vi "JSONconfig.vi"(2 "error in (no error)":errorcluster, 3 "file path (use dialog)":path, 4 "config file inputs":T5 {"Oscilloscope Configuration Input Array"."vertical coupling" items=["AC", "DC", "Ground"]}) -> (0 "error out":errorcluster, 1 "Instrument Configuration Clusters":T4 {"Oscilloscope Configuration Input Array"."vertical coupling" items=["AC", "DC", "Ground"]})   [LabVIEW 2019]
uses:
  Controls/VISA_power_Control.ctl
  Controls/RFBlockControl.ctl
  <instrlib>/niScope/Controls/niScope vertical coupling.ctl
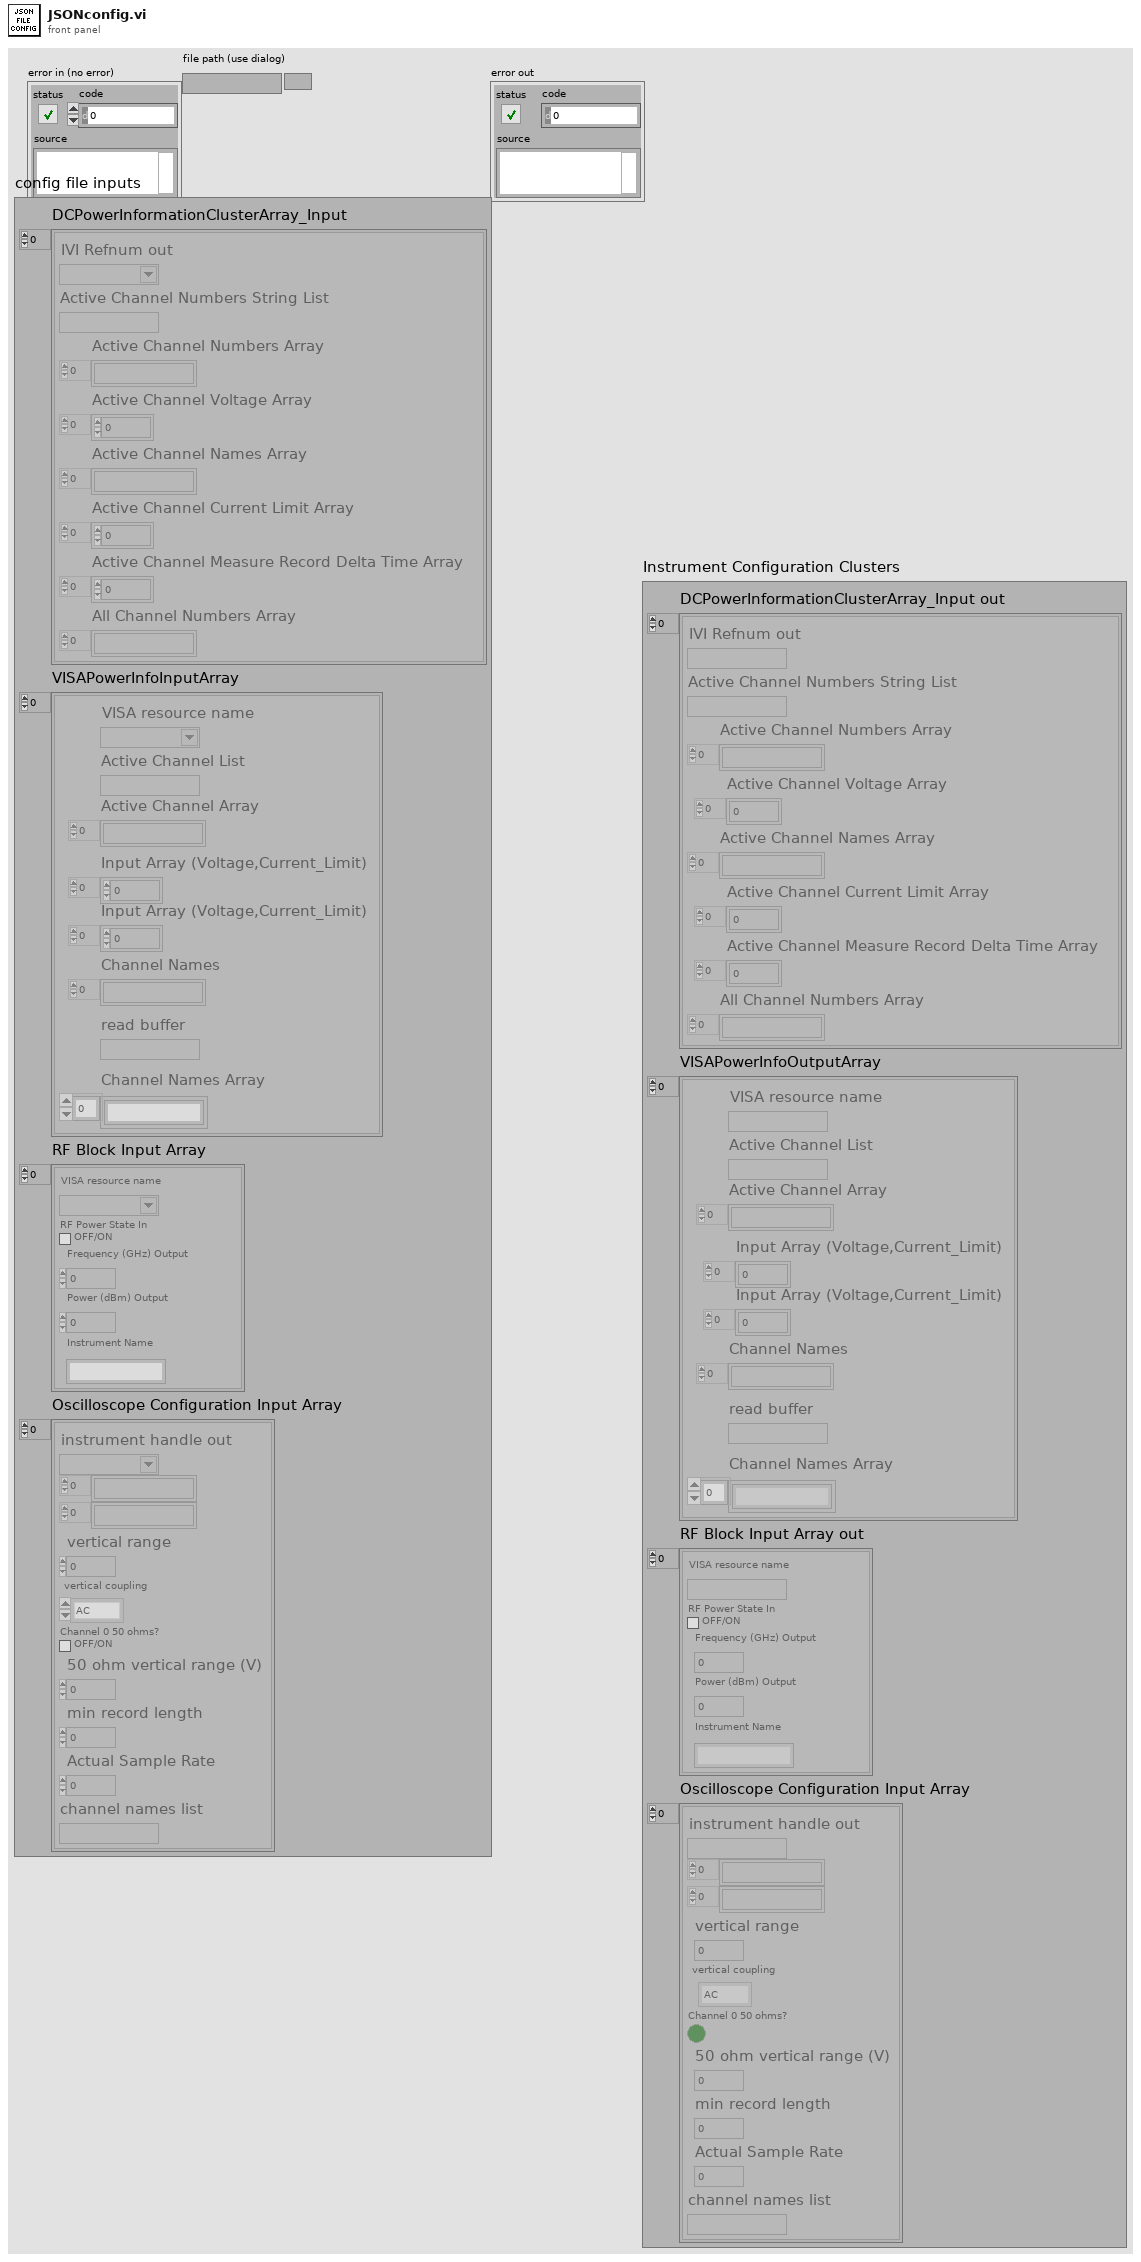
[diagram p1: front panel]
types:
  T1 = typedef "VISA_power_Control.ctl" = cluster{"VISA resource name":refnum<visa-resource-name>, "Active Channel List":string, "Active Channel Array":string[], "Input Array (Voltage,Current_Limit)":dbl[], "Input Array (Voltage,Current_Limit)":dbl[], "Channel Names":string[], "read buffer":string, "Channel Names Array":string[]}
  T2 = typedef "RFBlockControl.ctl" = cluster{"VISA resource name":refnum<visa-resource-name>, "RF Power State In":bool, "Frequency (GHz) Output":dbl, "Power (dBm) Output":dbl, "Instrument Name":string}
  T3 = typedef "niScope vertical coupling.ctl" = i32
  T4 = cluster{"DCPowerInformationClusterArray_Input out":cluster{"IVI Refnum out":refnum<k15>, "Active Channel Numbers String List":string, "Active Channel Numbers Array":string[], "Active Channel Voltage Array":dbl[], "Active Channel Names Array":string[], "Active Channel Current Limit Array":dbl[], "Active Channel Measure Record Delta Time Array":dbl[], "All Channel Numbers Array":string[]}[], "VISAPowerInfoOutputArray":T1[], "RF Block Input Array out":T2[], "Oscilloscope Configuration Input Array":cluster{"instrument handle out":refnum<k15>, string[], string[], "vertical range":dbl, "vertical coupling":T3, "Channel 0 50 ohms?":bool, "50 ohm vertical range (V)":dbl, "min record length":i32, "Actual Sample Rate":dbl, "channel names list":string}[]}
  T5 = cluster{"DCPowerInformationClusterArray_Input":cluster{"IVI Refnum out":refnum<k15>, "Active Channel Numbers String List":string, "Active Channel Numbers Array":string[], "Active Channel Voltage Array":dbl[], "Active Channel Names Array":string[], "Active Channel Current Limit Array":dbl[], "Active Channel Measure Record Delta Time Array":dbl[], "All Channel Numbers Array":string[]}[], "VISAPowerInfoInputArray":T1[], "RF Block Input Array":T2[], "Oscilloscope Configuration Input Array":cluster{"instrument handle out":refnum<k15>, string[], string[], "vertical range":dbl, "vertical coupling":T3, "Channel 0 50 ohms?":bool, "50 ohm vertical range (V)":dbl, "min record length":i32, "Actual Sample Rate":dbl, "channel names list":string}[]}
  T6 = cluster{"VISA resource name":refnum<visa-resource-name>, "String List":string, string[], "Input Array (Voltage,Current_Limit)":dbl[], "Input Array (Voltage,Current_Limit)":dbl[], "Channel Names":string[], "read buffer":string}
  T7 = enum16{"open", "replace", "create", "open or create", "replace or create", "replace or create with confirmation"}
  T8 = cluster{"IVI Refnum out":refnum<k15>, "Active Channel Numbers String List":string, "Active Channel Numbers Array":string[], "Active Channel Voltage Array":dbl[], "Active Channel Names Array":string[], "Active Channel Current Limit Array":dbl[], "Active Channel Measure Record Delta Time Array":dbl[], "All Channel Numbers Array":string[]}[]
  T9 = cluster{"instrument handle out":refnum<k15>, string[], string[], "vertical range":dbl, "vertical coupling":T3, "Channel 0 50 ohms?":bool, "50 ohm vertical range (V)":dbl, "min record length":i32, "Actual Sample Rate":dbl, "channel names list":string}[]
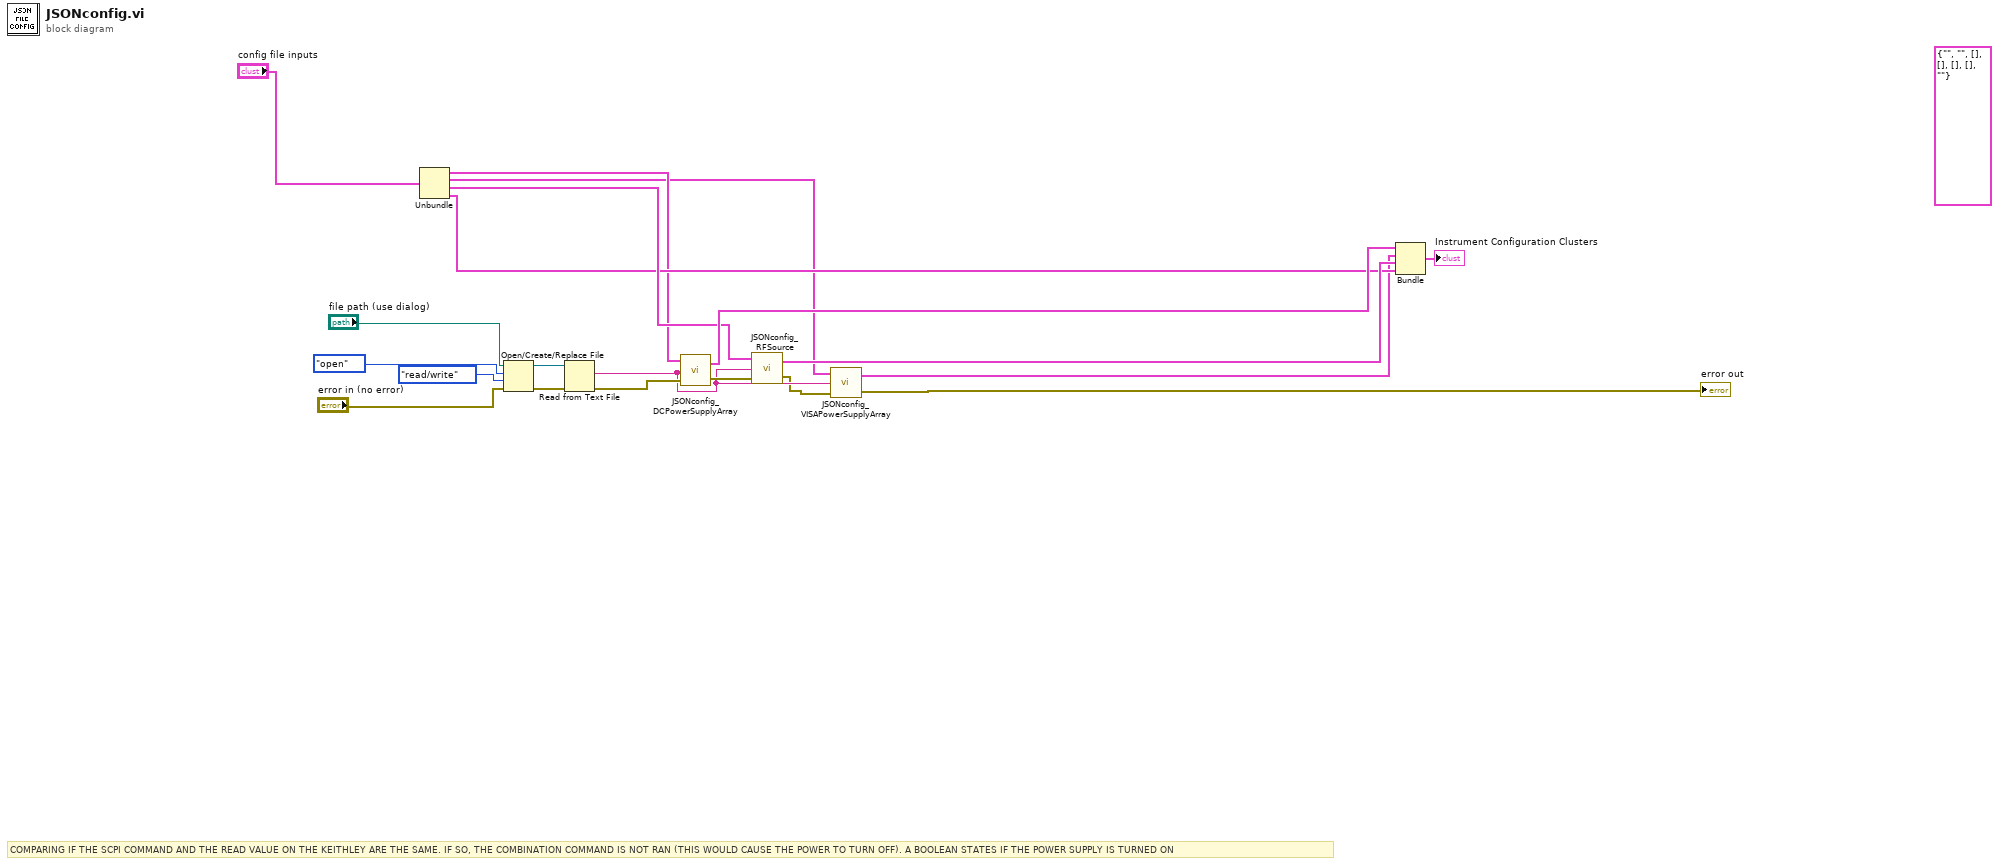
[diagram p0: block diagram]
diagram:
  (unwired) T6 {"VISA resource name"="", "String List"="", [], "Input Array (Voltage,Current_Limit)"=[], "Input Array (Voltage,Current_Limit)"=[], "Channel Names"=[], "read buffer"=""} ("element")
  # "COMPARING IF THE SCPI COMMAND AND THE READ VALUE ON THE KEITHLEY ARE THE SAME. IF SO, THE COMBINATION COMMAND IS NOT RAN (THIS WOULD CAUSE THE POWER TO TURN OFF). A BOOLEAN STATES IF THE POWER SUPPLY IS TURNED ON"
  n1 = Unbundle("config file inputs") -> ("DCPowerInformationClusterArray_Input"=w14:T8, "VISAPowerInfoInputArray"=w4:T1[], "RF Block Input Array"=w18:T2[], "Oscilloscope Configuration Input Array"=w16:T9)
  n2 = Open/Create/Replace File(file path (use dialog)="file path (use dialog)", error in="error in (no error)", operation (0:open)=T7."open", access (0:read/write)=enum16{"read/write", "read-only", "write-only"}."read/write") -> (refnum out=w11:refnum<file>, error out=w9:errorcluster)  [unwired: 2 in, 1 out]
  n3 = Read from Text File(file (use dialog)=w11, error in=w9) -> (text=w7:string, error out=w15:errorcluster)  [unwired: 2 in, 2 out]
  n4 = call "JSONconfig_DCPowerSupplyArray.vi"("error in (no error)"=w15, "String"=w7, "DCPowerInformationClusterArray_Input in"=w14) -> ("error out"=w17:errorcluster, "DCPowerInformationClusterArray_Input out"=w19:T8)
  n5 = call "JSONconfig_RFSource.vi"("error in (no error)"=w17, "String"=w7, "RF Block Input Array in"=w18) -> ("error out"=w6:errorcluster, "RF Block Input Array out"=w20:T2[])
  n6 = call "JSONconfig_VISAPowerSupplyArray.vi"("error in (no error)"=w6, "String"=w7, "VISAPowerInfoInputArray"=w4) -> ("error out"=→"error out":errorcluster, "VISAPowerInfoOutputArray"=w3:T1[])
  n7 = Bundle("DCPowerInformationClusterArray_Input out"=w19, "VISAPowerInfoOutputArray"=w3, "RF Block Input Array out"=w20, "Oscilloscope Configuration Input Array"=w16) -> (→"Instrument Configuration Clusters":T4)  [unwired: 1 in]
